vi "槽边合法性检查.vi"(9 "Caliper Results (check_AngleDistance)":sgl[][](array[numeric]) format="%.2f") -> (3 "槽核查通过":bool)   [LabVIEW 2015]
panel:
  in  "中心产品到槽口的角度":sgl
  in  "原始槽宽":sgl
  in  "槽两边夹角":sgl
  in  "限度-合理槽边间距-上限":dbl=15.0
  in  "限度-合理的槽边沿夹角-平行度":dbl=2.0
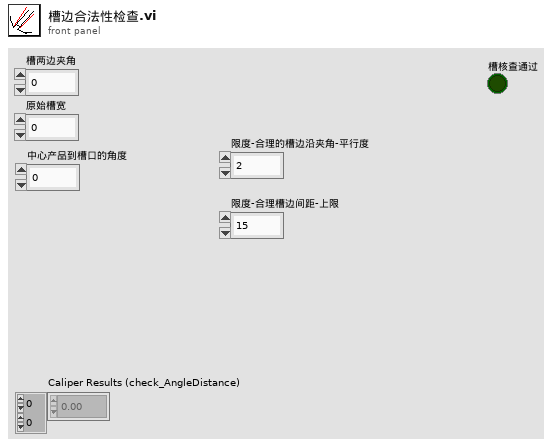
[diagram p1: front panel]
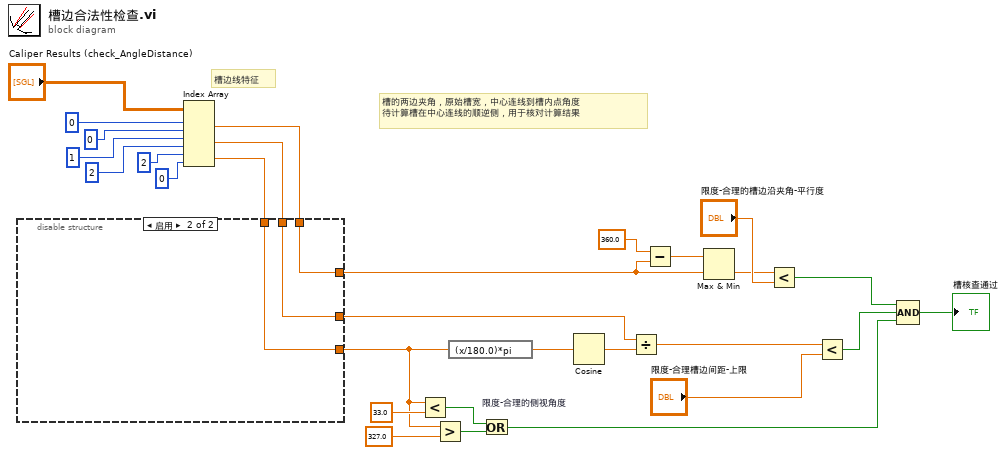
[diagram p0: block diagram]
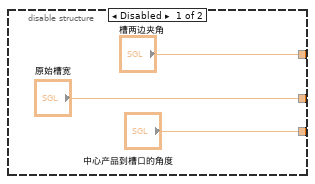
[diagram p2: hidden frame]
diagram:
  # "槽边线特征"
  # "槽的两边夹角，原始槽宽，中心连线到槽内点角度\n待计算槽在中心连线的顺逆侧，用于核对计算结果"
  n1 = Index Array(array="Caliper Results (check_AngleDistance)", index (row) #1=0 ("索引 (行)"), index (col) #1=0 ("禁用的索引 (列)"), index (row) #2=1 ("索引 (行)"), index (col) #2=2 ("禁用的索引 (列)"), index (row) #3=2 ("索引 (行)"), index (col) #3=0 ("禁用的索引 (列)")) -> (element #1=w3:sgl, element #2=w2:sgl, element #3=w1:sgl)
  n2 = disable-structure shown="启用" {
    disable-tunnel: ["槽两边夹角" w35] -> w14
    disable-tunnel: ["原始槽宽" w34] -> w13
    disable-tunnel: ["中心产品到槽口的角度" w33] -> w12
    disable-tunnel: w3 -> [_ w35]
    disable-tunnel: w2 -> [_ w34]
    disable-tunnel: w1 -> [_ w33]
    frame Disabled {
    }
    frame Enabled {
    }
  }
  n3 = Less?(x=w12, y=33.0) -> (x < y?=w16:bool)
  n4 = Greater?(x=w12, y=327.0) -> (0:w17:bool)
  n5 = expression code="(x/180.0)*pi" ("degrees to radians")(w12) -> (w29:sgl)
  n6 = Or "限度-合理的侧视角度"(x=w16, y=w17) -> (x .or. y?=w15:bool)
  n7 = Cosine(x=w29) -> (cos(x)=w28:sgl)
  n8 = Divide(x=w13, y=w28) -> (x/y=w20:sgl)
  n9 = Subtract(x=360.0, y=w14) -> (x-y=w26:dbl)
  n10 = Max & Min(x=w26, y=w14) -> (min(x,y)=w19:dbl)  [unwired: 1 out]
  n11 = Less?(x=w19, y="限度-合理的槽边沿夹角-平行度") -> (x < y?=w22:bool)
  n12 = Less?(x=w20, y="限度-合理槽边间距-上限") -> (x < y?=w21:bool)
  n13 = Compound Arithmetic op=AND ("复合运算")(w22, w21, w15) -> (→"槽核查通过":bool)
